vi "TrajectoryConfig_GetCentripetalAccelConstraint.vi"(11 "inTRAJECTORY_CONFIG":T1 {"End Velocity" format="%20.4f"; "StartVelocity" format="%20.4f"; "Max Acceleration" format="%20.4f"; "MaxVelocity" format="%20.4f"}) -> (1 "Constraint Exists":bool, 3 "Centripital Accleration Constraint":T2 {"Max Cent Accel" format="%20.4f"})   [LabVIEW 2019, in "Trajectory_Library.lvlib"]
doc: "Retrieves the Centripital Acceleration constraint from the Trajectory Configuration.\n\nNote: If more than once instance of the Centripital Accleration constraint exists only the first one is returned. (Only one of these should be defined.)\n\nParameters:\n - InTrajectoryConfig -- The trajectory configuration data structure\n\nReturns:\n - MaxCentAccel -- The data cluster, which contains the maximum centripetal acceleration (meters/sec^2)\n - Constraint Exists -- Returns TRUE if this constraint is defined in the trjaectory configuration."
uses:
  Trajectory_Library.lvlib
  <vilib>/Utility/Data Type/NI_Data Type.lvlib
  TypeDef/TRAJ_CONSTRAINT_CENTRIPETAL_ACCEL.ctl
  TypeDef/TRAJ_CONFIG.ctl
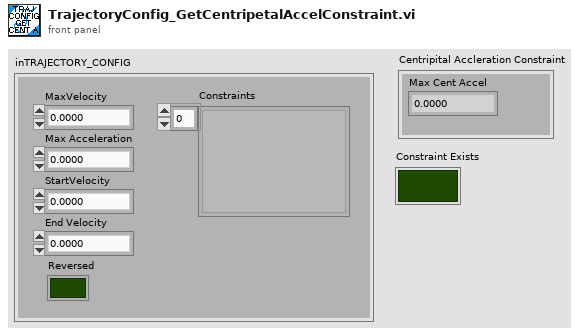
[diagram p1: front panel]
types:
  T1 = typedef "Trajectory_Library.lvlib/TRAJ_CONFIG.ctl" = cluster{"MaxVelocity":dbl, "Max Acceleration":dbl, "StartVelocity":dbl, "End Velocity":dbl, "Reversed":bool, "Constraints":variant[]}
  T2 = typedef "Trajectory_Library.lvlib/TRAJ_CONSTRAINT_CENTRIPETAL_ACCEL.ctl" = cluster{"Max Cent Accel":dbl}
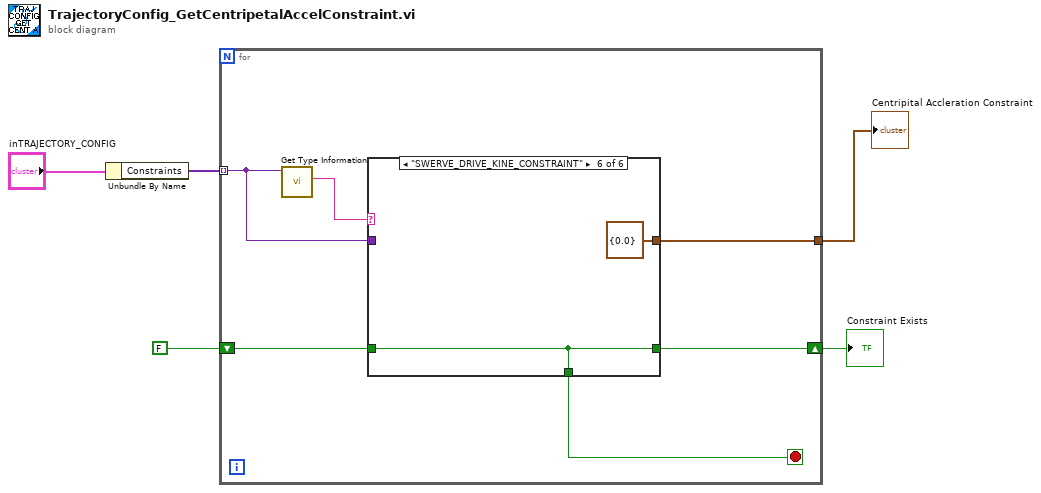
[diagram p0: block diagram]
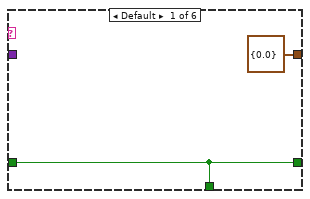
[diagram p2: hidden frame]
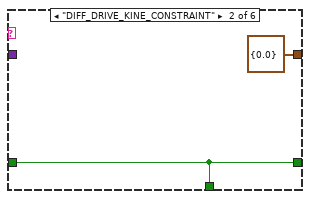
[diagram p3: hidden frame]
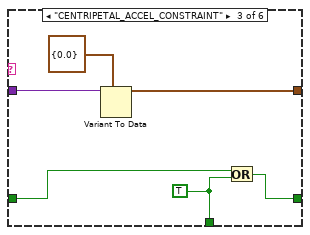
[diagram p4: hidden frame]
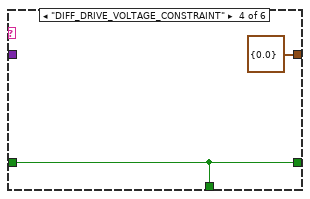
[diagram p5: hidden frame]
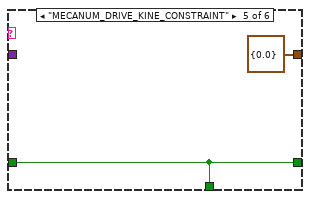
[diagram p6: hidden frame]
diagram:
  n1 = Unbundle By Name("inTRAJECTORY_CONFIG") -> ("Constraints"=w4:variant[])
  n2 = for {
    tunnel: w4 -> [w10] mode=indexing
    shift-right: [w8] -> w2
    shift-left: FALSE -> [w9]
    tunnel: [w7] -> w1
    stop <- w6 stop-if-true
    n3 = call <vilib>:"Get Type Information.vi"("variant"=w10) -> ("name"=w11:string)  [unwired: 6 in, 4 out]
    n4 = case shown="\"SWERVE_DRIVE_KINE_CONSTRAINT\"" w11 {
      tunnel: w10 -> [_ _ w20 _ _ _]
      tunnel: w9 -> [w13 w15 w17 w23 w25 w27]
      tunnel: [w13 w15 w18 w23 w25 w27] -> w8
      tunnel: [T2 {"Max Cent Accel"=0.0} ("CENTRIPETAL_ACCEL_CONSTRAINT") T2 {"Max Cent Accel"=0.0} ("CENTRIPETAL_ACCEL_CONSTRAINT") w19 T2 {"Max Cent Accel"=0.0} ("CENTRIPETAL_ACCEL_CONSTRAINT") T2 {"Max Cent Accel"=0.0} ("CENTRIPETAL_ACCEL_CONSTRAINT") T2 {"Max Cent Accel"=0.0} ("CENTRIPETAL_ACCEL_CONSTRAINT")] -> w7
      tunnel: [w13 w15 w16 w23 w25 w27] -> w6
      frame Default {
      }
      frame "DIFF_DRIVE_KINE_CONSTRAINT" {
      }
      frame "CENTRIPETAL_ACCEL_CONSTRAINT" {
        w16 = TRUE
        n5 = Variant To Data(type=T2 {"Max Cent Accel"=0.0} ("CENTRIPETAL_ACCEL_CONSTRAINT"), Variant=w20) -> (data=w19:T2)  [unwired: 1 in, 1 out]
        n6 = Or(x=w17, y=w16) -> (x .or. y?=w18:bool)
      }
      frame "DIFF_DRIVE_VOLTAGE_CONSTRAINT" {
      }
      frame "MECANUM_DRIVE_KINE_CONSTRAINT" {
      }
      frame "SWERVE_DRIVE_KINE_CONSTRAINT" {
      }
    }
  }
  "Centripital Accleration Constraint" <- w1
  "Constraint Exists" <- w2
